vi "resetError.vi"(8 "error in (no error)":errorcluster, 11 "BECHWCBasic in":refnum<class "BECHWCBasic.lvclass">) -> (0 "error out":errorcluster, 3 "BECHWCBasic out":refnum<class "BECHWCBasic.lvclass">)   [LabVIEW 2009, in "Hardware.lvlib" / "HWControllers.lvlib" / "BECHWCBasic.lvclass"]
uses:
  BECHWCBasic.lvclass
  HWController.lvclass
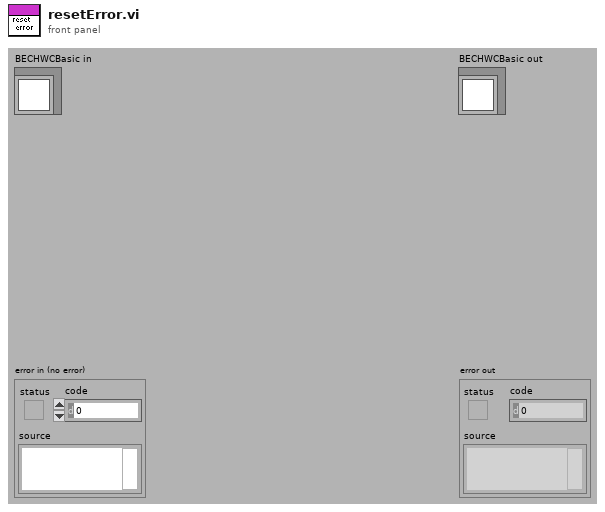
[diagram p1: front panel]
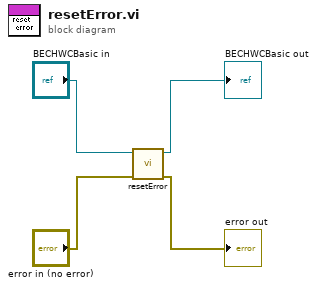
[diagram p0: block diagram]
diagram:
  n1 = call-parent "resetError.vi"("error in (no error)"="error in (no error)", "HWController in"="BECHWCBasic in") -> ("error out"=→"error out":errorcluster, "HWController out"=→"BECHWCBasic out":refnum<class "BECHWCBasic.lvclass">)  [unwired: 8 in]
